vi "SubVI.vi"(8 "error in":errorcluster, 11 "reference":refnum<vi>) -> (0 "error out":errorcluster, 3 "SubVI out":refnum<class "SubVI.lvclass">)   [LabVIEW 2014, in "SubVI.lvclass"]
uses:
  SubVI.lvclass
  Node/Node.lvclass
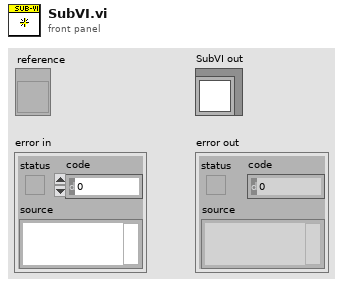
[diagram p1: front panel]
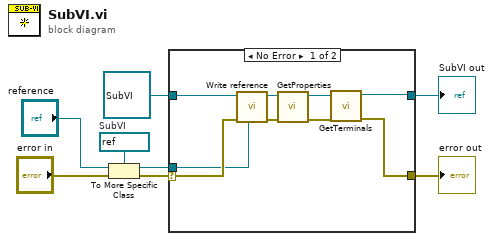
[diagram p0: block diagram]
diagram:
  w8 = refnum<vi> refnum  # SubVI
  n1 = To More Specific Class(target class=w8, reference="reference", error in="error in") -> (specific class reference=w5:refnum<vi>, error out=w6:errorcluster)
  n2 = case shown="No Error" w6 {
    selector: w6 -> [w17 w19]
    tunnel: w5 -> [w15 _]
    tunnel: refnum<class "SubVI.lvclass"> refnum ("SubVI in") -> [w16 w18]
    tunnel: [w11 w18] -> w1
    tunnel: [w9 w19] -> w2
    frame No Error {
      n3 = call-dynamic "Write reference.vi"("reference"=w15, "error in"=w17, "GObject in"=w16) -> ("error out"=w13:errorcluster, "GObject out"=w14:refnum<class "SubVI.lvclass">)  [unwired: 5 in]
      n4 = call-dynamic "GetProperties.vi"("error in"=w13, "SubVI in"=w14) -> ("error out"=w10:errorcluster, "SubVI out"=w12:refnum<class "SubVI.lvclass">)  [unwired: 8 in]
      n5 = call "GetTerminals.vi"("error in"=w10, "Node in"=w12) -> ("error out"=w9:errorcluster, "Node out"=w11:refnum<class "SubVI.lvclass">)  [unwired: 8 in]
    }
    frame Error {
    }
  }
  "error out" <- w2
  "SubVI out" <- w1
